vi "Read in TDMS.vi"(8 "error in (no error)":errorcluster, 11 "tdms in":refnum<k34>) -> (0 "error out":errorcluster, 1 "PI pos (um)":dbl[](array[numeric]), 2 "Timestamps (ms)":u64[](array[numeric]), 3 "tdms file out":refnum<k34>)   [LabVIEW 2020]
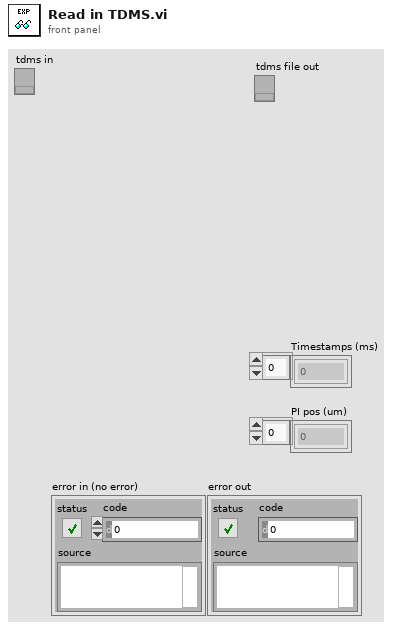
[diagram p1: front panel]
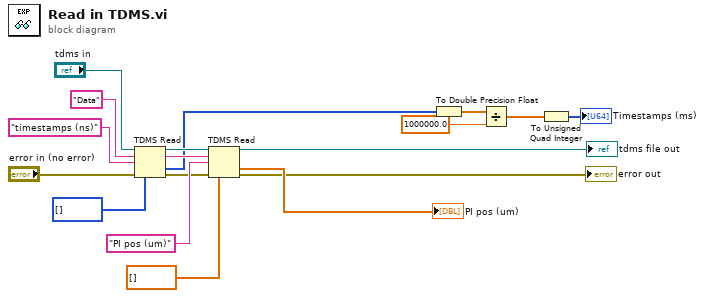
[diagram p0: block diagram]
diagram:
  n1 = TDMS Read(0:"tdms in", 5:"Data" ("group name in (Untitled)"), 7:"timestamps (ns)" ("group name in (Untitled)"), 11:"error in (no error)", 12:u64[] [] ("Timestamps (ms)")) -> (4:w12:refnum<k34>, 6:w16:string, 10:w5:u64[], 15:w13:errorcluster)  [unwired: 3 in, 2 out]
  n2 = TDMS Read(0:w12, 5:w16, 7:"PI pos (um)" ("group name in (Untitled)"), 11:w13, 12:dbl[] [] ("PI pos (um)")) -> (4:→"tdms file out":refnum<k34>, 10:→"PI pos (um)":dbl[], 15:→"error out":errorcluster)  [unwired: 3 in, 3 out]
  n3 = To Double Precision Float(number=w5) -> (double precision float=w3:dbl[])
  n4 = Divide(x=w3, y=1000000.0) -> (x/y=w2:dbl[])
  n5 = To Unsigned Quad Integer(1:w2) -> (0:→"Timestamps (ms)":u64[])
